vi "Stimulus.GetVersion.vi"(8 "error in (no error)":errorcluster, 10 "Exists":bool, 11 "Path":path) -> (0 "error out":errorcluster, 3 "Build":u32)   [LabVIEW 2015, in "Single Station Execution.lvlib"]
uses:
  Single Station Execution.lvlib
  NationalInstruments.VeriStand.RealTimeSequenceDefinitionApi
  NationalInstruments.VeriStand
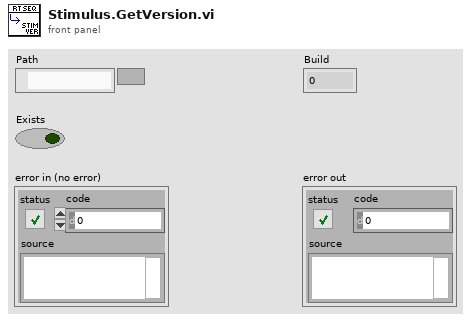
[diagram p1: front panel]
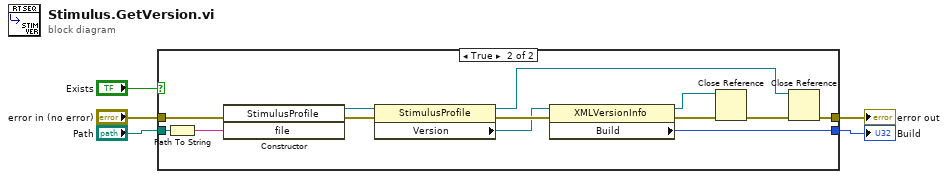
[diagram p0: block diagram]
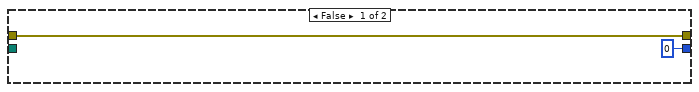
[diagram p2: hidden frame]
diagram:
  n1 = case shown="True" "Exists" {
    tunnel: "Path" -> [_ w14]
    tunnel: "error in (no error)" -> [w6 w10]
    tunnel: [w6 w13] -> w3
    tunnel: [u32 0 ("Build") w12] -> w5
    frame False {
    }
    frame True {
      n2 = Path To String(path=w14) -> (string=w11:string)
      n3 = constructor class="StimulusProfile"(error in=w10, "file"=w11) -> (reference out=w8:refnum<k24>, error out=w9:errorcluster)  [unwired: 2 in, 2 out]
      n4 = property class="StimulusProfile"(reference=w8, error in=w9) -> (reference out=w16:refnum<k24>, error out=w20:errorcluster, "Version"=w19:refnum<k24>)
      n5 = property class="XMLVersionInfo"(reference=w19, error in=w20) -> (reference out=w17:refnum<k24>, error out=w18:errorcluster, "Build"=w12:u32)
      n6 = Close Reference(reference=w17, error in (no error)=w18) -> (error out=w15:errorcluster)
      n7 = Close Reference(reference=w16, error in (no error)=w15) -> (error out=w13:errorcluster)
    }
  }
  "Build" <- w5
  "error out" <- w3
